vi "Start Module.vi"(8 "error in (no error)":errorcluster) -> (0 "error out":errorcluster, 3 "Module Running":bool)   [LabVIEW 2015, in "Generic Module Library.lvlib" / "Template G_Module.lvlib"]
uses:
  Template G_Module.lvlib
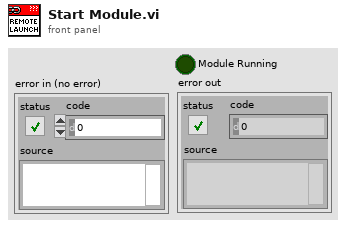
[diagram p1: front panel]
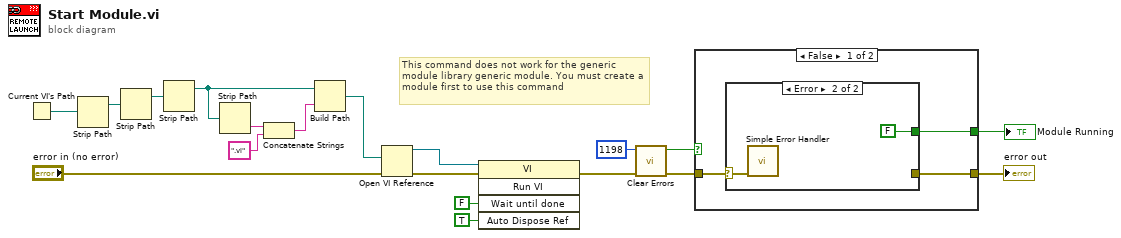
[diagram p0: block diagram]
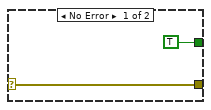
[diagram p2: hidden frame]
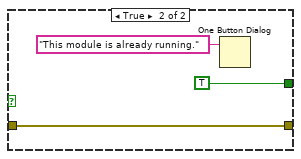
[diagram p3: hidden frame]
diagram:
  # "This command does not work for the generic module library generic module. You must create a module first to use this command"
  n1 = Current VI's Path() -> (path=w11:path)
  n2 = Strip Path(path=w11) -> (stripped path=w10:path)  [unwired: 1 out]
  n3 = Strip Path(path=w10) -> (stripped path=w9:path)  [unwired: 1 out]
  n4 = Strip Path(path=w9) -> (stripped path=w3:path)  [unwired: 1 out]
  n5 = Strip Path(path=w3) -> (name=w8:string)  [unwired: 1 out]
  n6 = Concatenate Strings(w8, ".vi" ("string")) -> (w2:string)
  n7 = Build Path(base path=w3, name or relative path=w2) -> (appended path=w5:path)
  n8 = Open VI Reference(vi path=w5, error in (no error)="error in (no error)") -> (vi reference=w4:refnum<vi>, error out=w6:errorcluster)  [unwired: 4 in]
  n9 = invoke class="VI" method="Run VI"(reference=w4, error in=w6, "Wait until done"=FALSE ("Wait Until Done"), "Auto Dispose Ref"=TRUE ("Auto Dispose Reference")) -> (error out=w18:errorcluster)  [unwired: 1 in, 4 out]
  n10 = call <vilib>:"Clear Errors.vi"("error in (no error)"=w18, "specific error code to clear (0: all)"=1198) -> ("error out"=w13:errorcluster, "specific error cleared?"=w14:bool)  [unwired: 4 in]
  n11 = case shown="False" w14 {
    tunnel: [w22 w29] -> w12
    tunnel: w13 -> [w21 w29]
    tunnel: [w20 TRUE] -> w1
    frame False {
      n12 = case shown="Error" w21 {
        selector: w21 -> [w24 w26]
        tunnel: [w24 _] -> w22
        tunnel: [TRUE FALSE] -> w20
        frame No Error {
        }
        frame Error {
          n13 = call <vilib>:"Simple Error Handler.vi"("error in (no error)"=w26) -> ()  [unwired: 4 in, 5 out]
        }
      }
    }
    frame True {
      n14 = One Button Dialog(message="This module is already running.") -> ()  [unwired: 1 in, 1 out]
    }
  }
  "error out" <- w12
  "Module Running" <- w1
